vi "ConvertImageToJpg.vi"(11 "buffer":string) -> (1 "image data":T1, 3 "new picture":picture)   [LabVIEW 2022 SP3]
uses:
  <vilib>/picture/picture.llb/imagedata.ctl
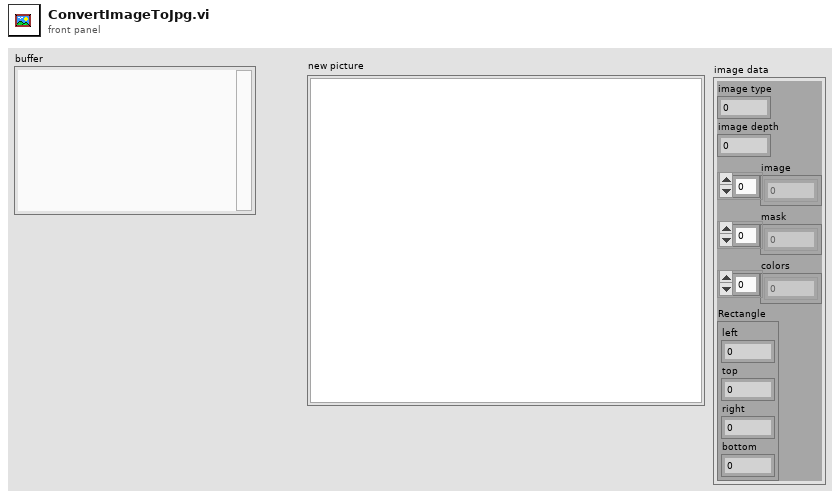
[diagram p1: front panel]
types:
  T1 = typedef "imagedata.ctl" = cluster{"image type":i32, "image depth":i32, "image":u8[], "mask":u8[], "colors":u32[], "Rectangle":cluster{"left":i16, "top":i16, "right":i16, "bottom":i16}}
  T2 = enum16{"big-endian, network order", "native, host order", "little-endian"}
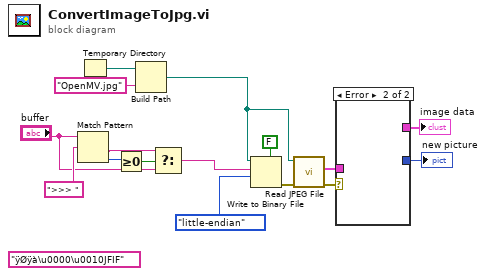
[diagram p0: block diagram]
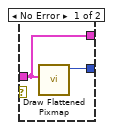
[diagram p2: hidden frame]
diagram:
  (unwired) "ÿØÿà\u0000\u0010JFIF"
  n1 = Match Pattern(string="buffer", regular expression=">>> ") -> (after substring=w3:string, offset past match=w5:i32)  [unwired: 1 in, 2 out]
  n2 = Temporary Directory() -> (w9:path)
  n3 = Greater Or Equal To 0?(x=w5) -> (x >= 0?=w4:bool)
  n4 = Build Path(base path=w9, name or relative path="OpenMV.jpg") -> (appended path=w7:path)
  n5 = Select(t=w3, s=w4, f="buffer") -> (s? t:f=w1:string)
  n6 = Write to Binary File(file (use dialog)=w7, data=w1, 5:FALSE ("prepend array or string size? (T)"), 9:T2."little-endian" ("byte order (0:big-endian, network order)")) -> (error out=w14:errorcluster)  [unwired: 2 in, 2 out]
  n7 = call <vilib>:"Read JPEG File.vi"("error in (no error)"=w14, "path to JPEG file"=w7) -> ("error out"=w10:errorcluster, "image data"=w13:T1)  [unwired: 7 in, 1 out]
  n8 = case shown="Error" w10 {
    tunnel: w13 -> [w17 _]
    tunnel: [w18 _] -> w12
    tunnel: [w17 _] -> w6
    frame No Error {
      n9 = call <vilib>:"Draw Flattened Pixmap.vi"("image data"=w17) -> ("new picture"=w18:picture)  [unwired: 8 in]
    }
    frame Error {
    }
  }
  "new picture" <- w12
  "image data" <- w6
